vi "AddressedToThisModule.vi"(10 "ModuleID":i32, 11 "ModuleAdmin In":refnum<class "ModuleAdmin.lvclass">) -> (1 "AddressedToAll (-1)":bool, 2 "AddressedToThisInstance?":bool, 3 "ModuleAdmin Out":refnum<class "ModuleAdmin.lvclass">)   [LabVIEW 2018, in "ModuleAdmin.lvlib"]
doc: "Determines if message is addressed to this module or all of the modules."
uses:
  ModuleAdmin.lvlib
  ModuleAdmin.lvclass
panel:
  out "Error Out":errorcluster
  in  "Error In":errorcluster
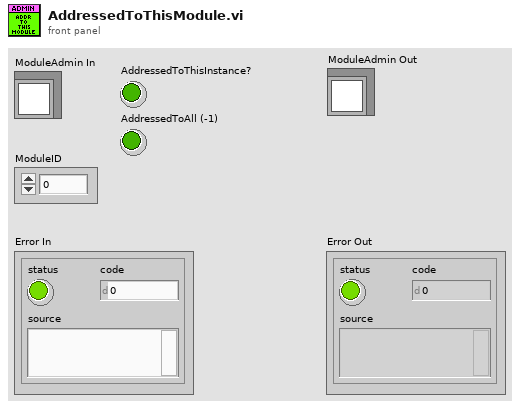
[diagram p1: front panel]
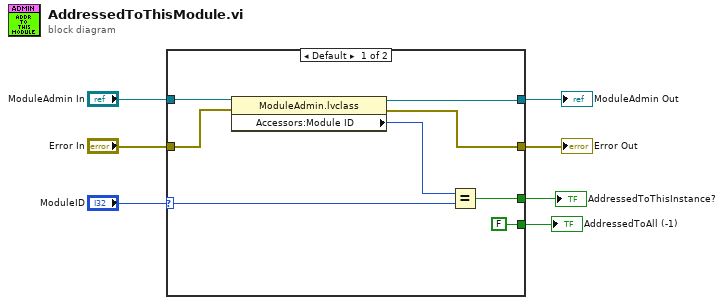
[diagram p0: block diagram]
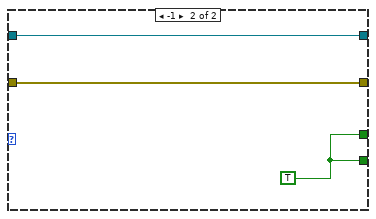
[diagram p2: hidden frame]
diagram:
  n1 = case shown="Default" "ModuleID" {
    selector: "ModuleID" -> [w13 _]
    tunnel: "ModuleAdmin In" -> [w15 w17]
    tunnel: [FALSE w18] -> w5
    tunnel: [w11 w18] -> w4
    tunnel: [w10 w16] -> w3
    tunnel: "Error In" -> [w9 w16]
    tunnel: [w8 w17] -> w1
    frame Default {
      n2 = property class="ModuleAdmin.lvclass"(reference=w15, error in=w9) -> (reference out=w8:refnum<class "ModuleAdmin.lvclass">, error out=w10:errorcluster, "Accessors:Module ID"=w14:i32)
      n3 = Equal?(x=w14, y=w13) -> (x = y?=w11:bool)
    }
    frame -1 {
      w18 = TRUE
    }
  }
  "AddressedToThisInstance?" <- w4
  "AddressedToAll (-1)" <- w5
  "Error Out" <- w3
  "ModuleAdmin Out" <- w1
